vi "Main.vi"() -> ()   [LabVIEW 2013]
panel:
  out "Bottom":dbl format="%.3f"
  out "Middle":dbl format="%.3f"
  out "Top":dbl format="%.3f"
  in  "XV-121":bool
  in  "N2CO2Switch 3":bool
  out "MFC-202-PV":dbl
  in  "MFC-202":dbl
  out "FeedRate":dbl
  in  "N2CO2Switch 2":bool
  in  "N2CO2Switch":bool
  out "Front Pannel":dbl[](graph)
  in  "Feeder Op":bool
  out "Balance":dbl
  in  "Auto Voltage":bool
  out "Steam Interlock":bool
  out "PI-201":dbl format="%#.1f"
  in  "XV-200":bool
  out "MFC-102 PV":dbl
  in  "MFC-102":dbl
  out "TI-322":dbl
  out "Boolean 4":bool
  out "MFC-201-PV":dbl
  in  "MFC-201":dbl
  in  "Steam":bool
  out "Estop":bool
  in  "Boolean":bool
  out "TI-632":dbl format="%.1f"
  in  "VLS Valves":bool=TRUE
  out "TI-603":dbl format="%.1f"
  in  "RESET":bool
  out "PI-501":dbl format="%.1f"
  out "TI-201":dbl format="%.1f"
  out "TI-640":dbl format="%.1f"
  out "TI-630":dbl format="%.1f"
  out "TI-622":dbl format="%.1f"
  out "TI-611":dbl format="%.1f"
  out "TI-503":dbl format="%.1f"
  out "TI-500E":dbl format="%.1f"
  out "TI-500C":dbl format="%.1f"
  out "TI-500A":dbl format="%.1f"
  out "TI-151":dbl format="%.1f"
  in  "XV-641":bool
  in  "XV-202":bool
  in  "XV-102":bool
  in  "XV-640":bool
  in  "XV-630":bool
  in  "XV-201":bool
  in  "XV-131":bool
  in  "XV-111":bool
  in  "MFC-111":dbl
  in  "MFC-101":dbl
  out "PI-421":dbl format="%.1f"
  out "PI-411":dbl format="%.1f"
  out "TI-501":dbl format="%.1f"
  out "PI-131":dbl format="%.1f"
  out "FAF1":bool
  out "TI-620":dbl format="%.1f"
  out "TI-502":dbl format="%.1f"
  in  "HX-500":bool
  in  "TI-530 2":dbl
  in  "TI-520 2":dbl
  in  "TI-510 2":dbl
  out "TI-530":dbl format="%.1f"
  out "TI-520":dbl format="%.1f"
  out "TI-510":dbl format="%.1f"
  in  "E-STOP\nButton":bool
  out "AFE":bool
  out "AFE3":bool
  out "AFE2":bool
  out "AFE1":bool
  in  "FT-310":dbl
  out "PI-641":dbl format="%.1f"
  out "TI-641":dbl format="%.1f"
  out "FI-641":dbl format="%.1f"
  in  "FT-410":dbl
  in  "FT-420":dbl
  out "TI-631":dbl format="%.1f"
  out "PI-621":dbl format="%.1f"
  out "TI-621":dbl format="%.1f"
  out "TI-610":dbl format="%.1f"
  out "AF":bool
  out "V-600 O2":dbl format="%.1f"
  out "TI-602":dbl format="%.1f"
  out "PI-600":dbl format="%.1f"
  out "TI-601":dbl format="%.1f"
  out "TI-600":dbl format="%.1f"
  out "Ash KO 1":bool
  out "Ash KO 3":bool
  out "Ash KO 2":bool
  out "AKOE":bool
  out "Waveform Chart 2":T1(graph)
  out "TI-321":dbl format="%.1f"
  out "TI-331":dbl format="%.1f"
  out "PI-321":dbl format="%.1f"
  out "TI-341":dbl format="%.1f"
  out "MFC-111-PV":dbl format="%.4f"
  in  "XV-101":bool
  out "MFC-101-PV":dbl format="%.4f"
  out "1 LO":bool
  out "1 HI":bool
  out "2 LO":bool
  out "2 HI":bool
  out "FAFE":bool
  out "Feed DP":dbl format="%.1f"
  out "V-200 O2":dbl format="%.1f"
  out "Feed Hopper":dbl(slide) scale=75.0..100.0
  out "PI-151":dbl format="%.1f"
  in  "Chiller":bool
  out "TI-642":dbl format="%.1f"
  in  "PCV-641":dbl format="%.2f"
  out "PCV-641 PV":dbl format="%.2f"
  out "AF 1":bool
  out "FAF":bool
  out "TI-342":dbl
  out "XV-201 IL":bool
  # "Supply:"
  # "HX-340"
  # "HX-330"
  # "Return:"
  # "SiC Skin Temps"
  # "Power KVA"
  # "Feeder"
  # "E-STOP\nIndicator"
  # "Argon"
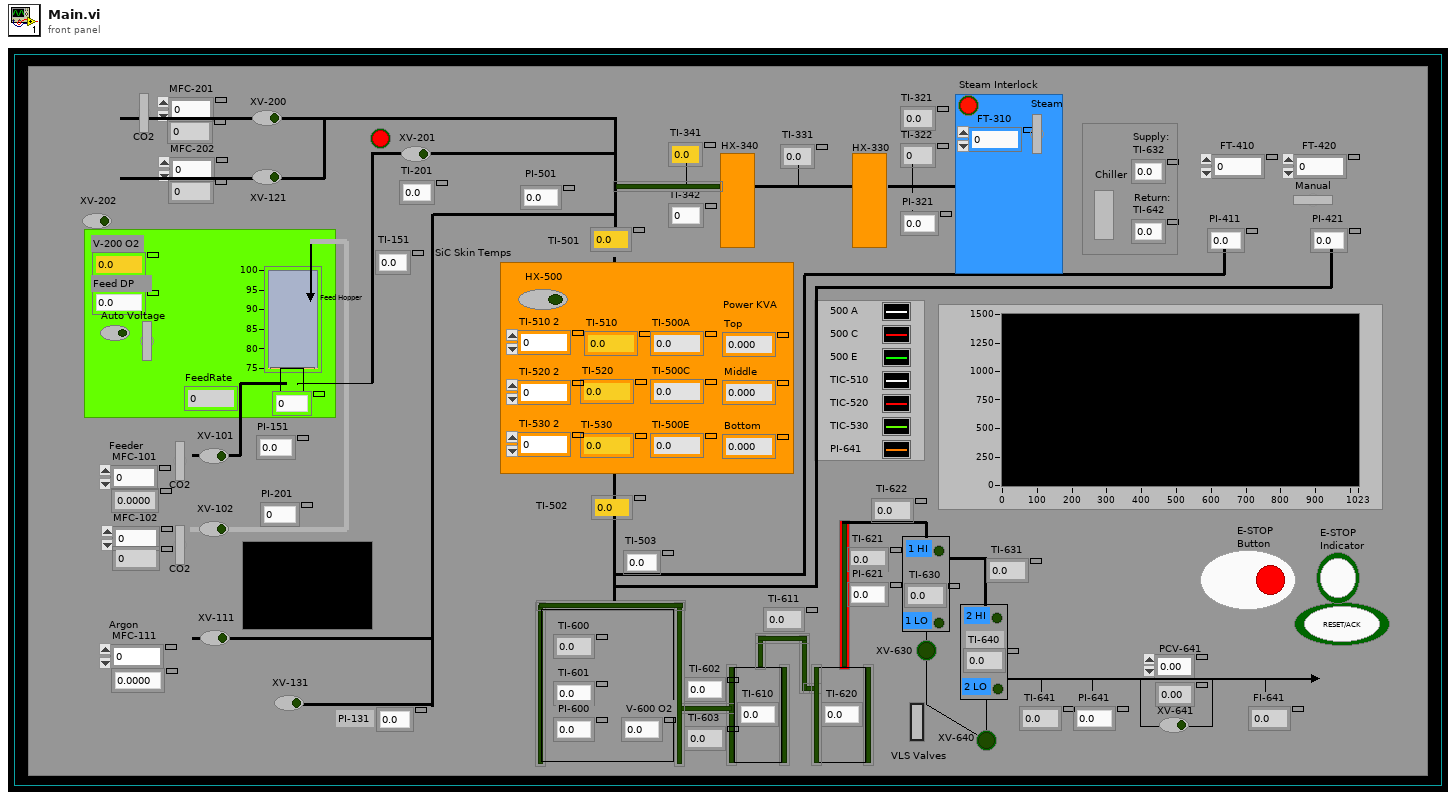
[diagram p1: front panel]
types:
  T1 = cluster{"[0]":dbl, "[1]":dbl, "[2]":dbl, "[3]":dbl, "[4]":dbl, "[5]":dbl, "[6]":dbl, "[7]":dbl, "[8]":dbl}
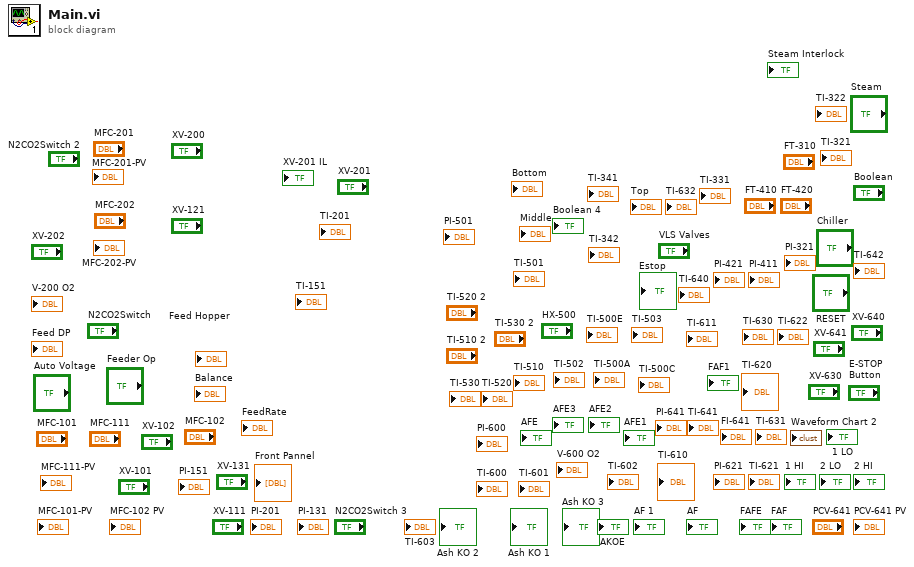
[diagram p0: block diagram]
diagram:
